vi "Get UI VI Reference.vi"(8 "error in (no error)":errorcluster, 11 "Single Computer PvP in":refnum<class "Single Computer PvP.lvclass">) -> (0 "error out":errorcluster, 2 "VI Refnum":refnum<vi>, 3 "Single Computer PvP out":refnum<class "Single Computer PvP.lvclass">)   [LabVIEW 2017, in "Single Computer PvP.lvclass"]
uses:
  Single Computer PvP.lvclass
  User Interface.vi
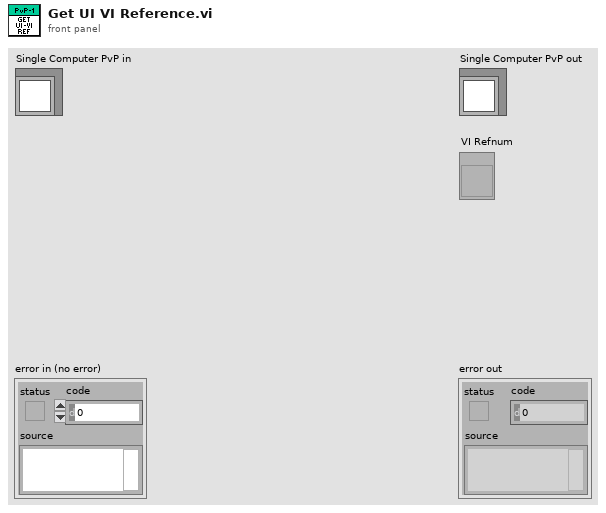
[diagram p1: front panel]
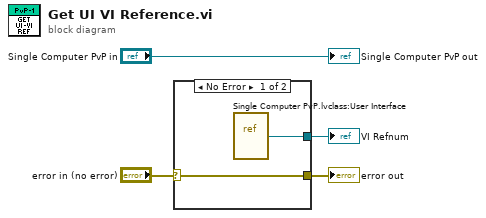
[diagram p0: block diagram]
diagram:
  n1 = case shown="No Error" "error in (no error)" {
    selector: "error in (no error)" -> [w5 w7]
    tunnel: [w5 w7] -> w2
    tunnel: [w6 _] -> w1
    frame No Error {
      n2 = vi-ref "Single Computer PvP.lvclass:User Interface.vi"() -> (w6:refnum<vi>)
    }
    frame Error {
    }
  }
  "error out" <- w2
  "VI Refnum" <- w1
  "Single Computer PvP out" <- "Single Computer PvP in"
